vi "Phase array Simulation(21.09.30_KJS).vi"() -> ()   [LabVIEW 2017]
uses:
  <vilib>/Analysis/3filter.llb/Filter Passband Type.ctl
  <vilib>/Analysis/baseanly.llb/Unit Vector (DBL).vi
  <vilib>/Analysis/2dsp.llb/Real FFT.vi
  <vilib>/Analysis/3filter.llb/FIR Windowed Filter (DBL).vi
  <vilib>/Analysis/NI_AALBase.lvlib
  <vilib>/Analysis/NI_AALPro.lvlib
panel:
  out "XY 그래프":cluster{dbl[], dbl[]}(graph)
  out "최대값":dbl
  in  "SNR(dB)":dbl=6.0
  out "doppler frequency % 2":dbl
  out "SUM signal(LPF)":waveform(dbl)(graph)
  out "S1+S3 signal(LPF)":waveform(dbl)(graph)
  out "S0+S2 signal(LPF)":waveform(dbl)(graph)
  out "Mixer(S1 +S3)":waveform(dbl)(graph)
  out "Mixer(S0 +S2)":waveform(dbl)(graph)
  out "S1+S3 FFT":waveform(dbl)(graph)
  out "S0+S2 FFT":waveform(dbl)(graph)
  out "S1+S3 signal":waveform(dbl)(graph)
  out "S0 +S2 signal":waveform(dbl)(graph)
  out "크기":i32
  in  "X(+)":bool
  in  "Delay time.A.1(sec)":dbl=0.5
  in  "Sampling frequency(Hz)":dbl=3000000.0
  in  "Pulse length(sec)":dbl=0.5
  in  "Amplitude(Vpeak)":dbl=1.0
  in  "Frequency(Hz)":dbl=614000.0
  in  "Carrier Frequency(Hz)":dbl=574000.0
  in  "S1+S3 Carrier Phsae":dbl=-90.0
  in  "S0+S2 Carrier Phsae":dbl=90.0
  in  "S0 Phsae":dbl=90.0
  in  "S1 Phsae":dbl=-90.0
  in  "S2 Phsae":dbl=-180.0
  in  "S3 Phsae":dbl=-270.0
  out "doppler frequency %":dbl
  in  "signal Dopphler On":bool
  in  "DpF":dbl=10000.0
  in  "Carrier Dopphler On":bool
  # "Signal Modeling Setting"
  # "Doppler shift Modeling Variable"
  # "Phase Modeling Variable"
  # "Simulation Button"
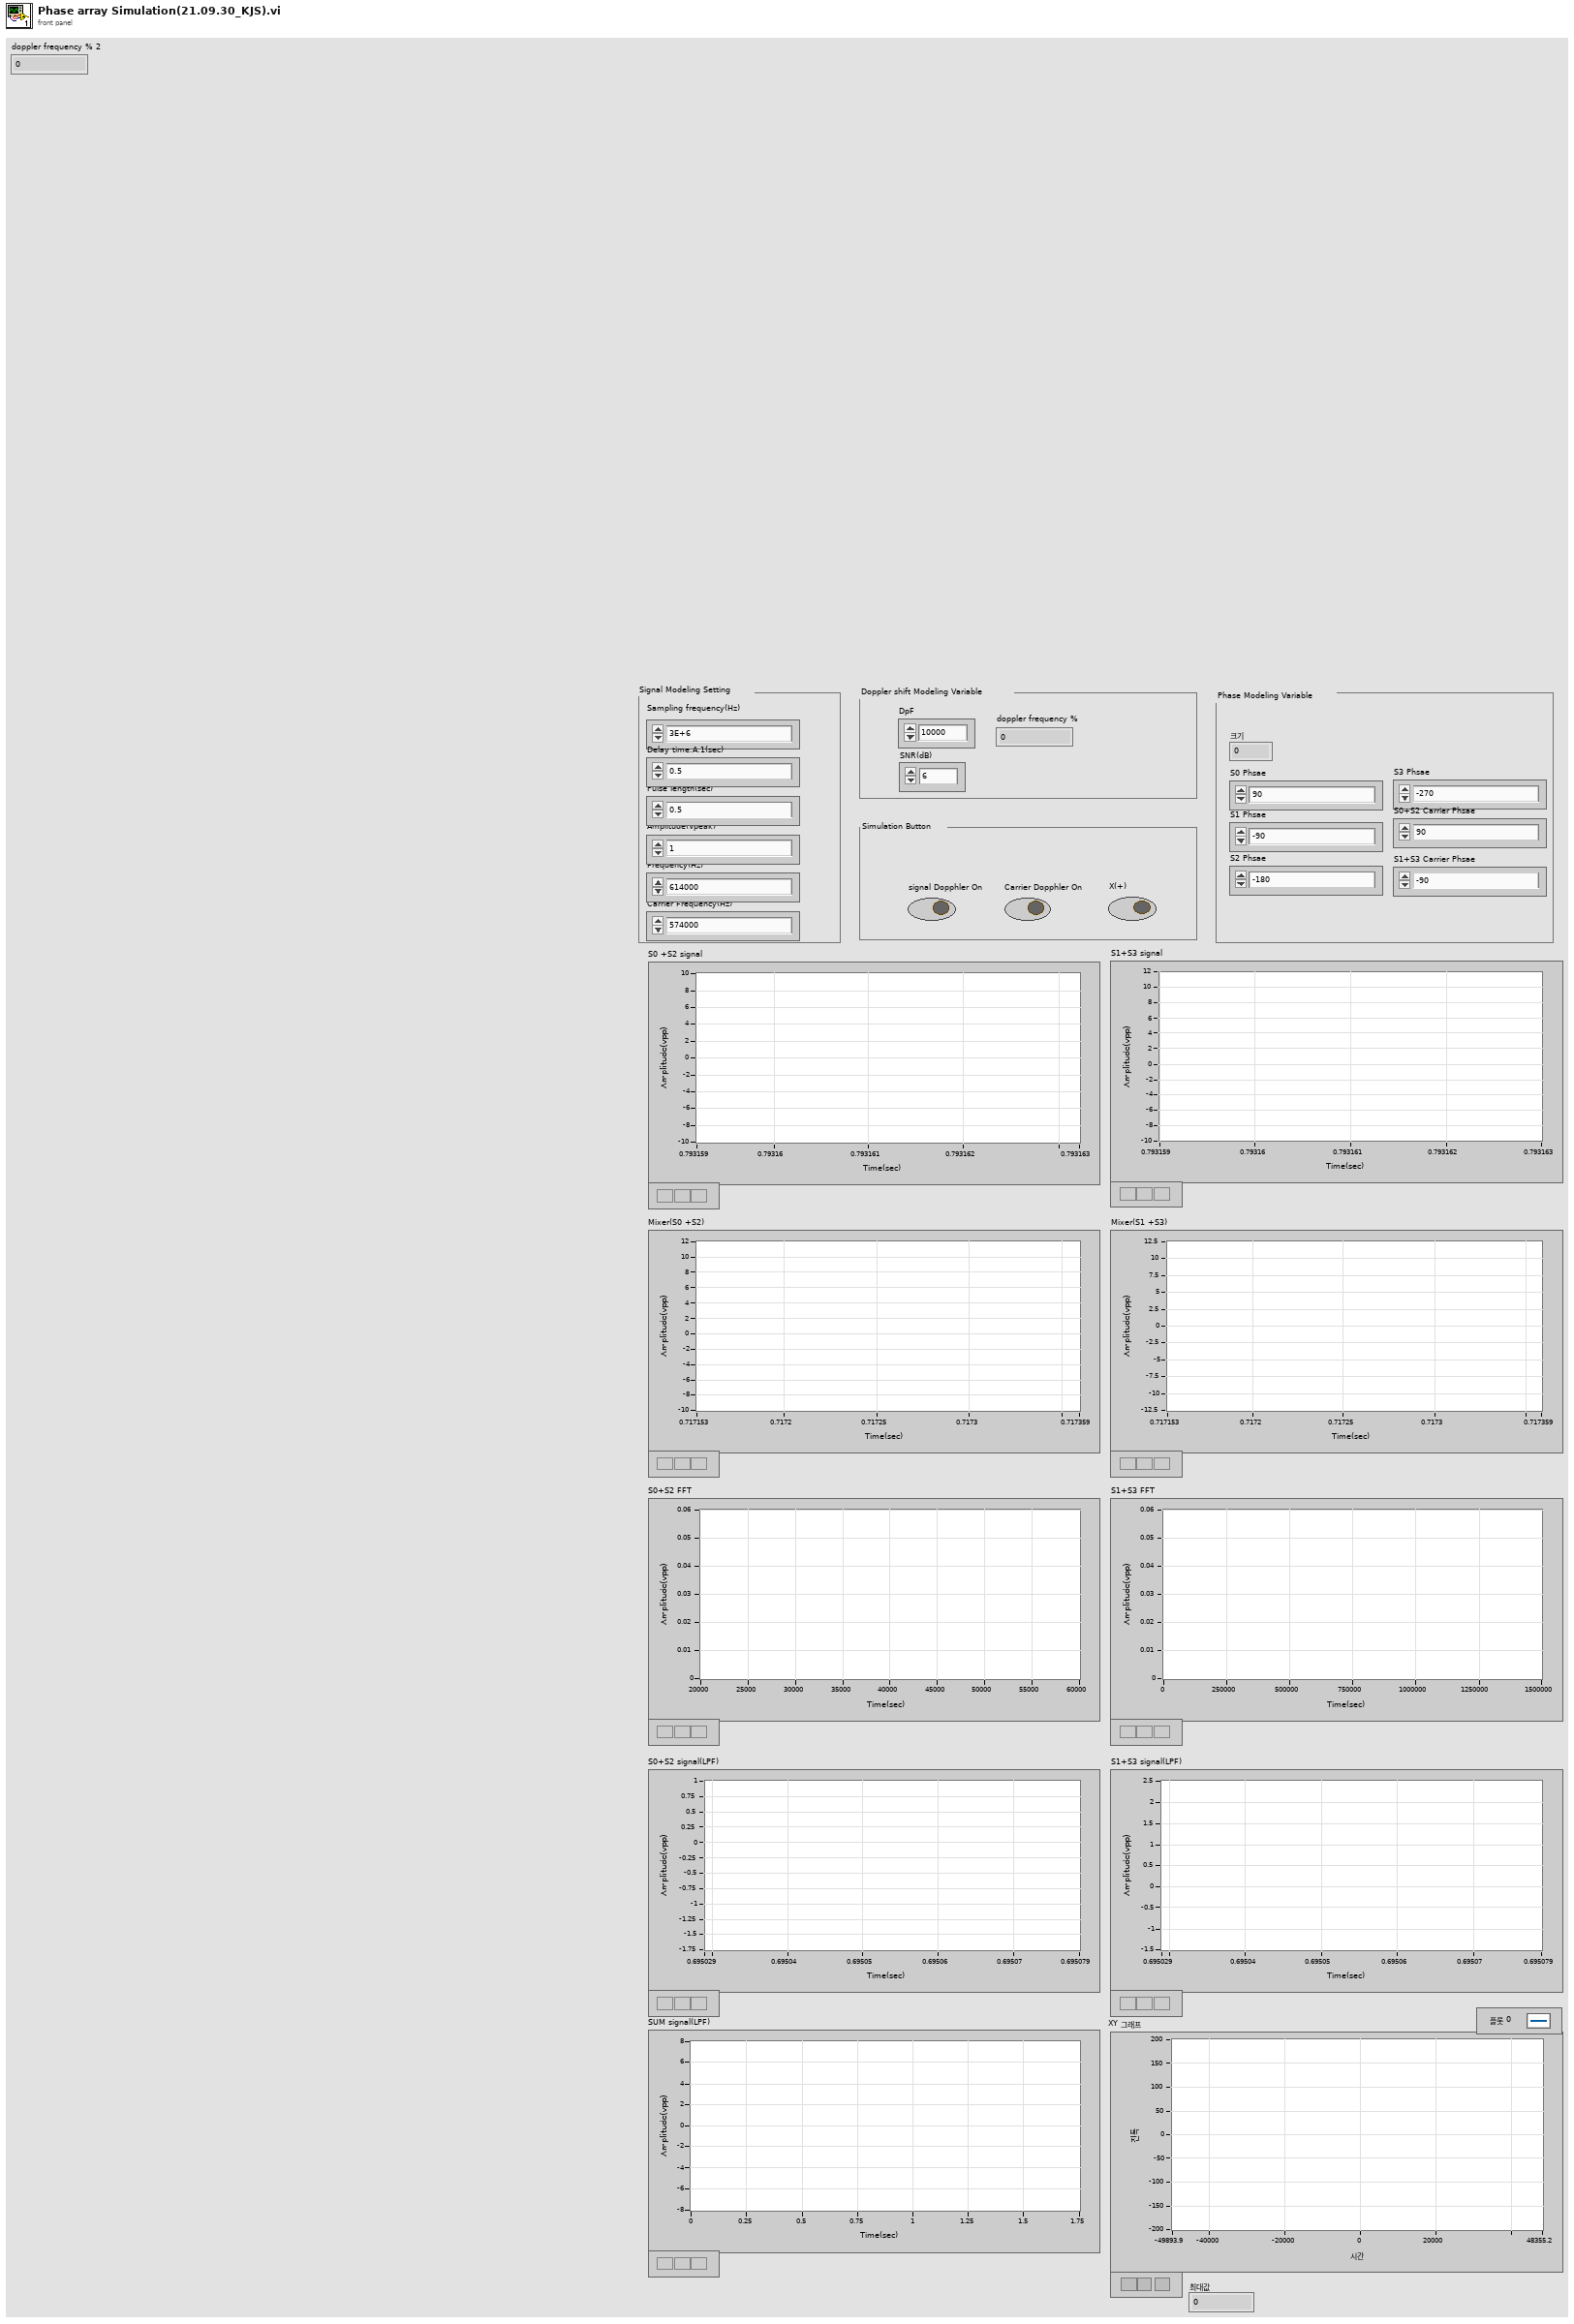
[diagram p1: front panel]
types:
  T1 = typedef "NI_AALBase.lvlib/Filter Passband Type.ctl" = enum32{"Lowpass", "Highpass", "Bandpass", "Bandstop"}
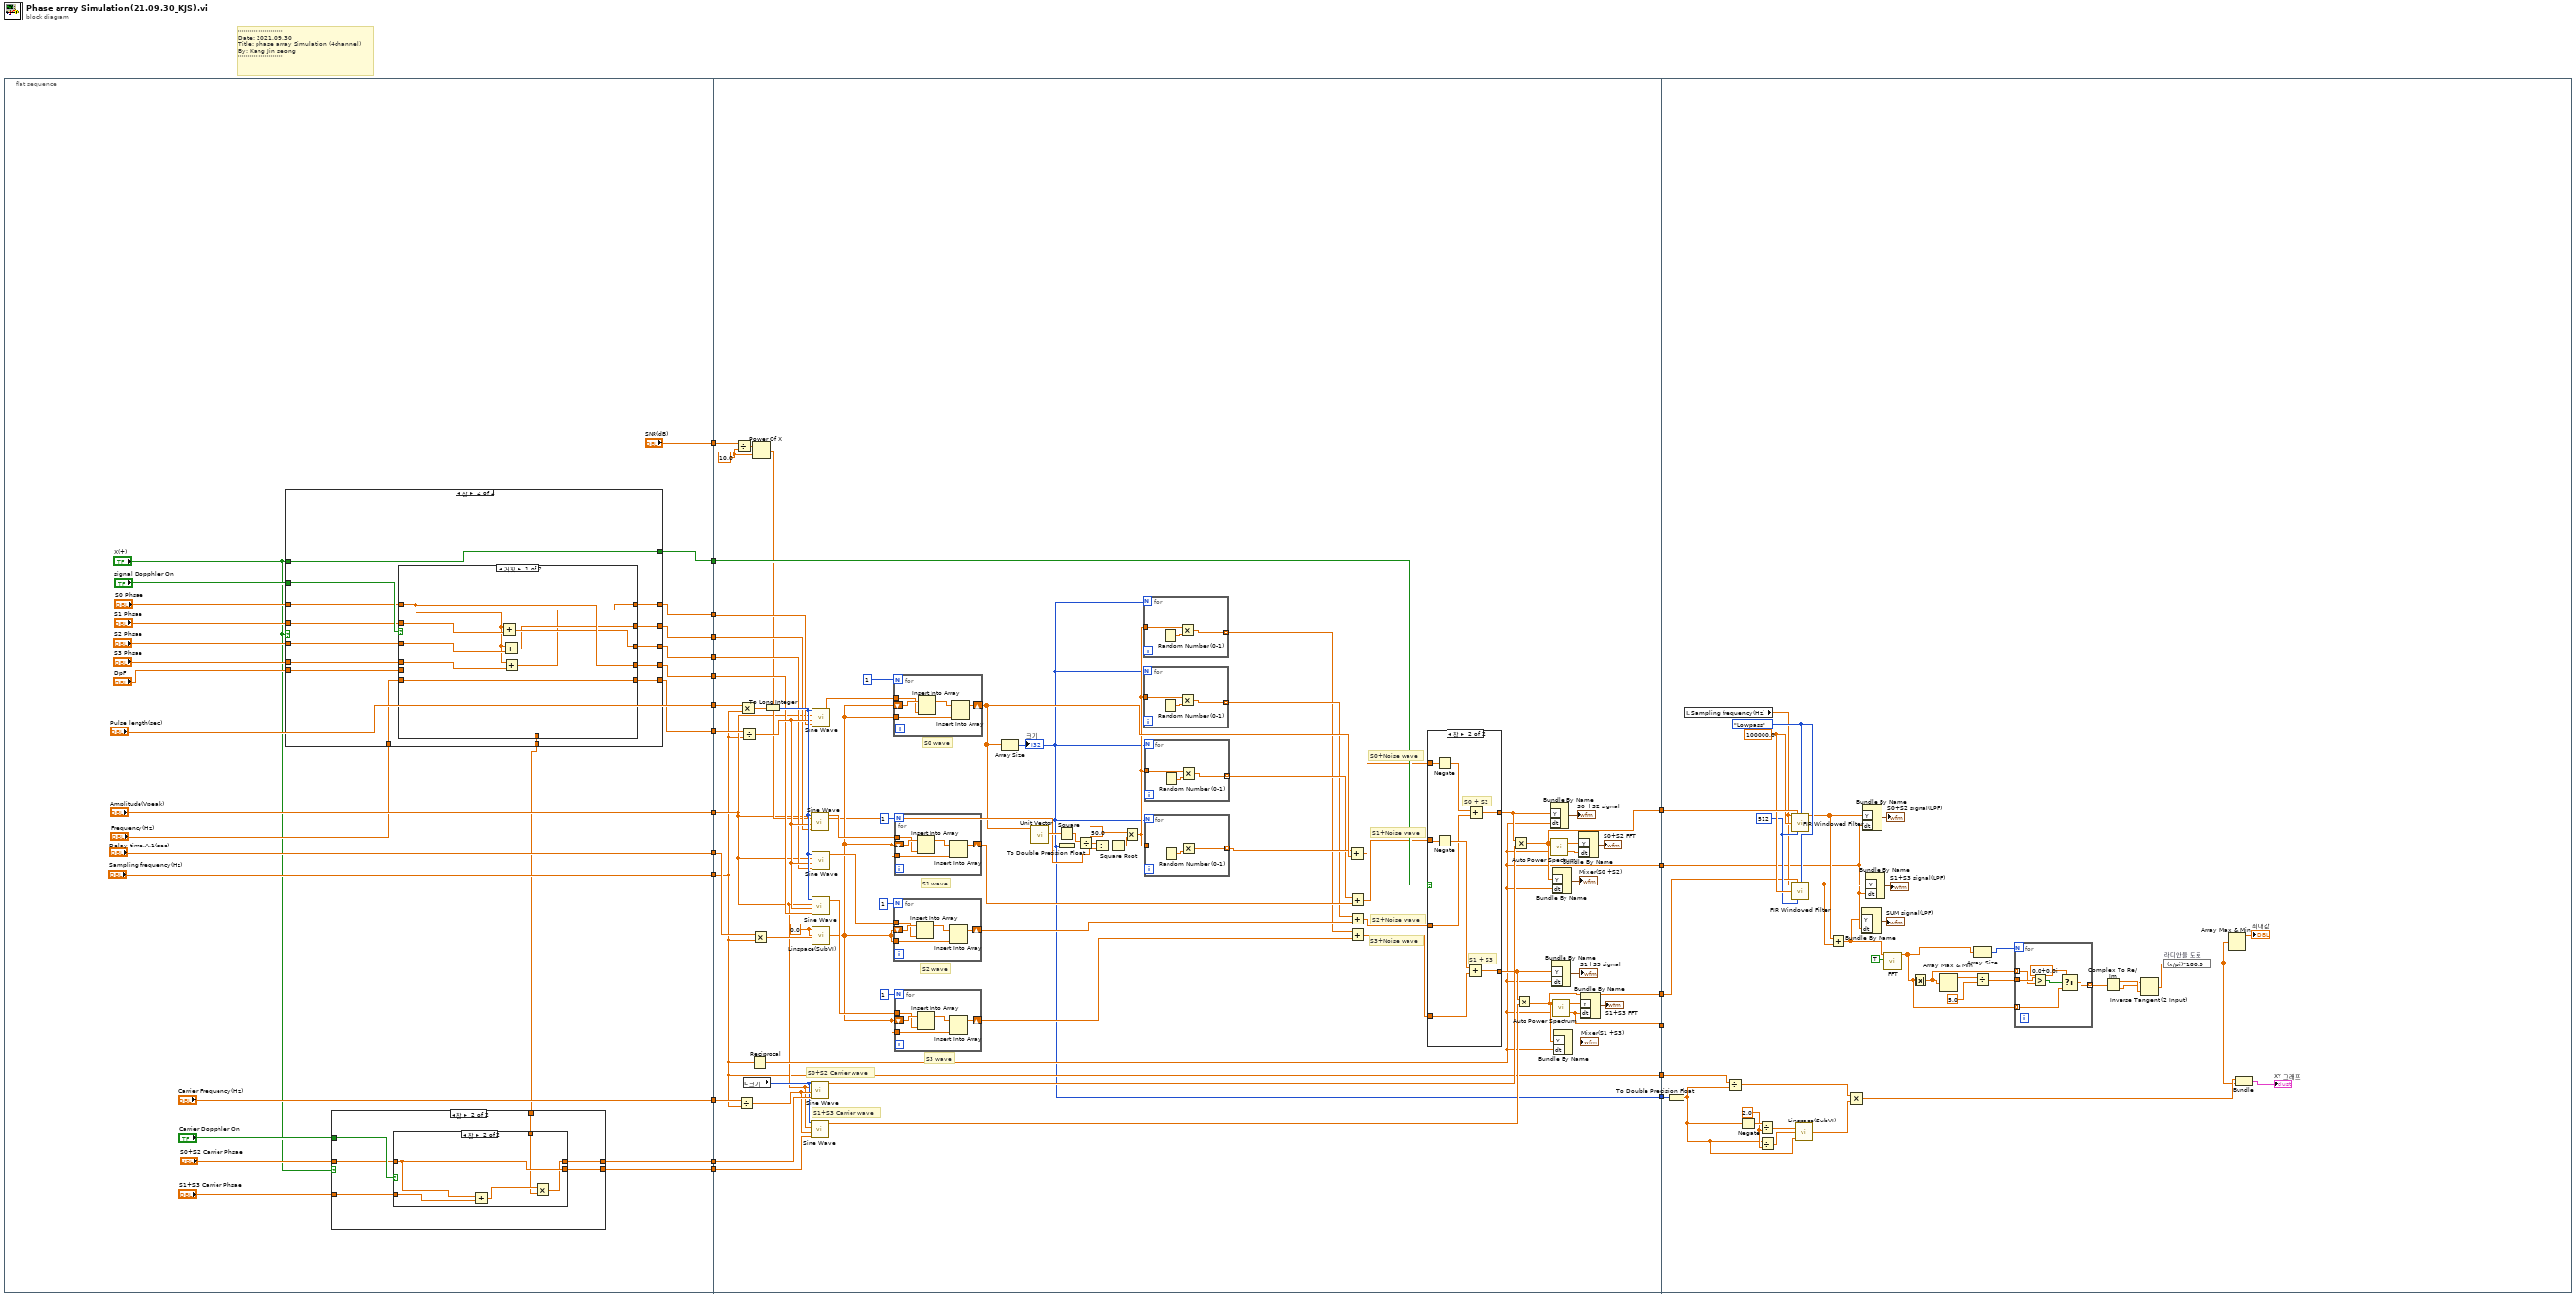
[diagram p0: block diagram]
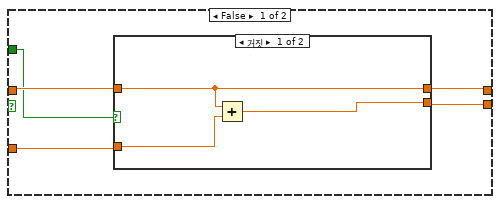
[diagram p2: hidden frame]
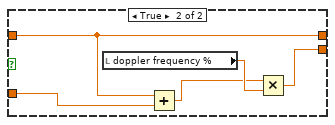
[diagram p3: hidden frame]
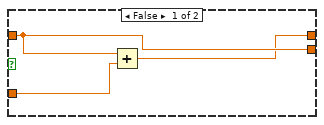
[diagram p4: hidden frame]
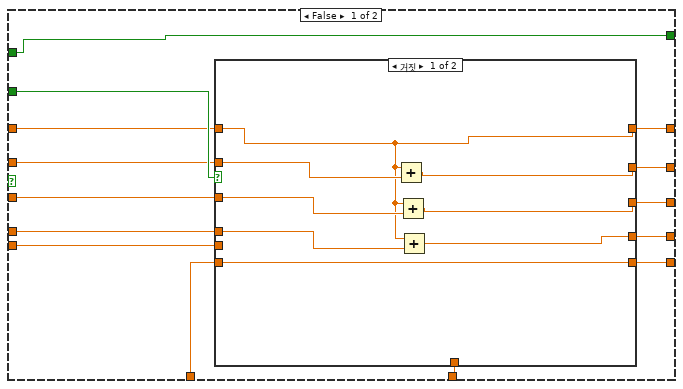
[diagram p5: hidden frame]
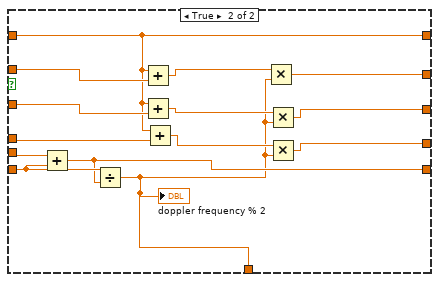
[diagram p6: hidden frame]
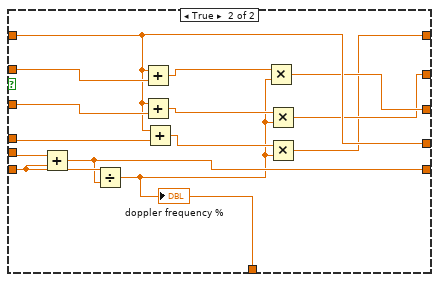
[diagram p7: hidden frame]
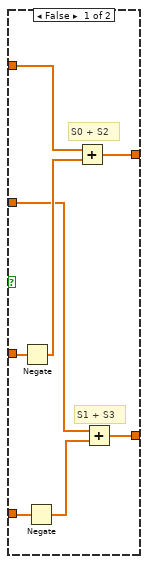
[diagram p8: hidden frame]
diagram:
  # "'''''''''''''''''''''''\nDate: 2021.09.30\nTitle: phase array Simulation (4channel)\nBy: Kang Jin seong\n'''''''''''''''''''''''"
  n1 = flat-sequence {
    tunnel: ["Carrier Frequency(Hz)"] -> w20
    tunnel: [w32] -> w19
    tunnel: ["Amplitude(Vpeak)"] -> w18
    tunnel: ["Pulse length(sec)"] -> w17
    tunnel: ["Sampling frequency(Hz)"] -> w16
    tunnel: ["Delay time.A.1(sec)"] -> w15
    tunnel: [w37] -> w14
    tunnel: [w36] -> w13
    tunnel: [w35] -> w12
    tunnel: [w34] -> w11
    tunnel: [w26] -> w10
    tunnel: [w25] -> w9
    tunnel: [w24] -> w5
    tunnel: ["SNR(dB)"] -> w4
    tunnel: w20 -> [w195]
    tunnel: w19 -> [w202]
    tunnel: w18 -> [w149]
    tunnel: w17 -> [w201]
    tunnel: w16 -> [w147]
    tunnel: w15 -> [w200]
    tunnel: w14 -> [w199]
    tunnel: w13 -> [w198]
    tunnel: w12 -> [w197]
    tunnel: w11 -> [w196]
    tunnel: w10 -> [w194]
    tunnel: w9 -> [w190]
    tunnel: [w178] -> w8
    tunnel: [w177] -> w7
    tunnel: [w176] -> w6
    tunnel: w5 -> [w175]
    tunnel: w4 -> [w172]
    tunnel: [w148] -> w3
    tunnel: [w147] -> w2
    tunnel: [w146] -> w1
    tunnel: w8 -> [w301]
    tunnel: w7 -> [w297]
    tunnel: w6 -> [w290]
    tunnel: w3 -> [_]
    tunnel: w2 -> [w277]
    tunnel: w1 -> [w276]
    frame #0 {
      n2 = case shown="참" "X(+)" {
        tunnel: "signal Dopphler On" -> [w86 w123]
        tunnel: "S0 Phsae" -> [w85 w122]
        tunnel: "S1 Phsae" -> [w84 w121]
        tunnel: "S2 Phsae" -> [w81 w120]
        tunnel: "S3 Phsae" -> [w80 w119]
        tunnel: [w79 w118] -> w37
        tunnel: [w78 w117] -> w36
        tunnel: [w77 w116] -> w35
        tunnel: [w76 w115] -> w34
        tunnel: "Frequency(Hz)" -> [w82 w114]
        tunnel: [w75 w113] -> w32
        tunnel: "DpF" -> [w83 w112]
        tunnel: [w87 w111] -> w24
        tunnel: "X(+)" -> [w87 w111]
        tunnel: [w74 w110] -> w21
        frame False {
          n3 = case shown="거짓" w86 {
            tunnel: w85 -> [w90 w99]
            tunnel: w84 -> [w94 w103]
            tunnel: w81 -> [w92 w101]
            tunnel: w80 -> [w89 w98]
            tunnel: [w90 w99] -> w79
            tunnel: [w93 w107] -> w78
            tunnel: [w91 w106] -> w77
            tunnel: [w88 w105] -> w76
            tunnel: w82 -> [w95 w108]
            tunnel: [w95 w104] -> w75
            tunnel: w83 -> [_ w109]
            tunnel: [_ w96] -> w74
            frame False {
              n4 = Add(x=w90, y=w94) -> (x+y=w93:dbl)
              n5 = Add(x=w90, y=w92) -> (x+y=w91:dbl)
              n6 = Add(x=w90, y=w89) -> (x+y=w88:dbl)
            }
            frame True {
              n7 = Add(x=w109, y=w108) -> (x+y=w104:dbl)
              n8 = Divide(x=w108, y=w104) -> (x/y=w96:dbl)
              "doppler frequency % 2" <- w96
              n9 = Add(x=w99, y=w103) -> (x+y=w102:dbl)
              n10 = Add(x=w99, y=w101) -> (x+y=w100:dbl)
              n11 = Add(x=w99, y=w98) -> (x+y=w97:dbl)
              n12 = Multiply(x=w102, y=w96) -> (x*y=w107:dbl)
              n13 = Multiply(x=w100, y=w96) -> (x*y=w106:dbl)
              n14 = Multiply(x=w97, y=w96) -> (x*y=w105:dbl)
            }
          }
        }
        frame True {
          n15 = case shown="거짓" w123 {
            tunnel: w122 -> [w127 w136]
            tunnel: w121 -> [w130 w142]
            tunnel: w120 -> [w129 w140]
            tunnel: w119 -> [w128 w138]
            tunnel: [w124 w133] -> w118
            tunnel: [w125 w134] -> w117
            tunnel: [w126 w135] -> w116
            tunnel: [w127 w136] -> w115
            tunnel: w114 -> [w131 w144]
            tunnel: [w131 w143] -> w113
            tunnel: w112 -> [_ w145]
            tunnel: [_ w132] -> w110
            frame False {
              n16 = Add(x=w127, y=w130) -> (x+y=w126:dbl)
              n17 = Add(x=w127, y=w129) -> (x+y=w125:dbl)
              n18 = Add(x=w127, y=w128) -> (x+y=w124:dbl)
            }
            frame True {
              n19 = Add(x=w145, y=w144) -> (x+y=w143:dbl)
              n20 = Divide(x=w144, y=w143) -> (x/y=w132:dbl)
              "doppler frequency %" <- w132
              n21 = Add(x=w136, y=w142) -> (x+y=w141:dbl)
              n22 = Add(x=w136, y=w140) -> (x+y=w139:dbl)
              n23 = Add(x=w136, y=w138) -> (x+y=w137:dbl)
              n24 = Multiply(x=w141, y=w132) -> (x*y=w135:dbl)
              n25 = Multiply(x=w139, y=w132) -> (x*y=w134:dbl)
              n26 = Multiply(x=w137, y=w132) -> (x*y=w133:dbl)
            }
          }
        }
      }
      n27 = case shown="참" "X(+)" {
        tunnel: "Carrier Dopphler On" -> [w47 w65]
        tunnel: "S0+S2 Carrier Phsae" -> [w51 w64]
        tunnel: "S1+S3 Carrier Phsae" -> [w50 w63]
        tunnel: [w49 w62] -> w26
        tunnel: [w48 w61] -> w25
        tunnel: w21 -> [_ w60]
        frame False {
          n28 = case shown="거짓" w47 {
            tunnel: w51 -> [w52 w55]
            tunnel: w50 -> [w54 w57]
            tunnel: [w52 w55] -> w49
            tunnel: [w53 w58] -> w48
            frame False {
              n29 = Add(x=w52, y=w54) -> (x+y=w53:dbl)
            }
            frame True {
              n30 = local read "doppler frequency %"() -> (w59:dbl)
              n31 = Add(x=w55, y=w57) -> (x+y=w56:dbl)
              n32 = Multiply(x=w56, y=w59) -> (x*y=w58:dbl)
            }
          }
        }
        frame True {
          n33 = case shown="참" w65 {
            tunnel: w64 -> [w67 w71]
            tunnel: w63 -> [w68 w73]
            tunnel: [w66 w70] -> w62
            tunnel: [w67 w71] -> w61
            tunnel: w60 -> [_ w69]
            frame False {
              n34 = Add(x=w67, y=w68) -> (x+y=w66:dbl)
            }
            frame True {
              n35 = Add(x=w71, y=w73) -> (x+y=w72:dbl)
              n36 = Multiply(x=w72, y=w69) -> (x*y=w70:dbl)
            }
          }
        }
      }
    }
    frame #1 {
      w174 = 10.0 ("y")
      w213 = 0.0 ("Start")
      # "S3+Noise wave"
      # "S2+Noise wave"
      # "S1+Noise wave"
      # "S0+Noise wave"
      # "S1+S3 Carrier wave"
      # "S0+S2 Carrier wave"
      # "S3 wave"
      # "S2 wave"
      # "S1 wave"
      # "S0 wave"
      n37 = Divide(x=w172, y=w174) -> (x/y=w173:dbl)
      n38 = Divide(x=w195, y=w147) -> (x/y=w191:dbl)
      n39 = Multiply(x=w201, y=w147) -> (x*y=w216:dbl)
      n40 = Divide(x=w202, y=w147) -> (x/y=w214:dbl)
      n41 = local read "크기"() -> (w150:i32)
      n42 = Reciprocal(x=w147) -> (1/x=w176:dbl)
      n43 = Multiply(x=w200, y=w147) -> (x*y=w212:dbl)
      n44 = Power Of X(1:w174, 2:w173) -> (0:w164:dbl)
      n45 = To Long Integer(number=w216) -> (32bit integer=w215:i32)
      n46 = call <vilib>:"Sine Wave.vi"("samples"=w150, "amplitude"=w149, "frequency"=w191, "phase in"=w194) -> ("sine wave"=w188:dbl[])  [unwired: 1 in, 2 out]
      n47 = call <vilib>:"Sine Wave.vi"("samples"=w215, "amplitude"=w149, "frequency"=w214, "phase in"=w198) -> ("sine wave"=w208:dbl[])  [unwired: 1 in, 2 out]
      n48 = call <vilib>:"Sine Wave.vi"("samples"=w150, "amplitude"=w149, "frequency"=w191, "phase in"=w190) -> ("sine wave"=w186:dbl[])  [unwired: 1 in, 2 out]
      n49 = call <vilib>:"Sine Wave.vi"("samples"=w215, "amplitude"=w149, "frequency"=w214, "phase in"=w196) -> ("sine wave"=w204:dbl[])  [unwired: 1 in, 2 out]
      n50 = call <vilib>:"Sine Wave.vi"("samples"=w215, "amplitude"=w149, "frequency"=w214, "phase in"=w199) -> ("sine wave"=w210:dbl[])  [unwired: 1 in, 2 out]
      n51 = call <vilib>:"Sine Wave.vi"("samples"=w215, "amplitude"=w149, "frequency"=w214, "phase in"=w197) -> ("sine wave"=w206:dbl[])  [unwired: 1 in, 2 out]
      n52 = call "Linspace(SubVI).vi"("NumElements"=w212, "End"=w213, "Start"=w213) -> ("Array"=w203:dbl[])
      n53 = for {
        N: 1 -> [_]
        shift-right: [w260] -> w163
        shift-left: w203 -> [w264]
        tunnel: w210 -> [w263]
        tunnel: w203 -> [w261]
        n54 = Insert Into Array(array=w264, new element=w263) -> (w262:dbl[])  [unwired: 1 in]
        n55 = Insert Into Array(array=w262, new element=w261) -> (w260:dbl[])  [unwired: 1 in]
      }
      n56 = for {
        N: 1 -> [_]
        shift-right: [w250] -> w161
        shift-left: w203 -> [w254]
        tunnel: w206 -> [w253]
        tunnel: w203 -> [w251]
        n57 = Insert Into Array(array=w254, new element=w253) -> (w252:dbl[])  [unwired: 1 in]
        n58 = Insert Into Array(array=w252, new element=w251) -> (w250:dbl[])  [unwired: 1 in]
      }
      n59 = for {
        N: 1 -> [_]
        shift-right: [w255] -> w162
        shift-left: w203 -> [w259]
        tunnel: w208 -> [w258]
        tunnel: w203 -> [w256]
        n60 = Insert Into Array(array=w259, new element=w258) -> (w257:dbl[])  [unwired: 1 in]
        n61 = Insert Into Array(array=w257, new element=w256) -> (w255:dbl[])  [unwired: 1 in]
      }
      n62 = for {
        N: 1 -> [_]
        shift-right: [w245] -> w160
        shift-left: w203 -> [w249]
        tunnel: w204 -> [w248]
        tunnel: w203 -> [w246]
        n63 = Insert Into Array(array=w249, new element=w248) -> (w247:dbl[])  [unwired: 1 in]
        n64 = Insert Into Array(array=w247, new element=w246) -> (w245:dbl[])  [unwired: 1 in]
      }
      n65 = Array Size(array=w163) -> (size(s)=w146:i32)
      "크기" <- w146
      n66 = call-poly <vilib>:"Unit Vector.vi"("Input Vector"=w163) -> ("norm"=w171:dbl)  [unwired: 8 in, 2 out]
      n67 = Square(x=w171) -> (x^2=w170:dbl)
      n68 = To Double Precision Float(number=w146) -> (double precision float=w169:dbl)
      n69 = Divide(x=w170, y=w169) -> (x/y=w168:dbl)
      n70 = Divide(x=w168, y=w164) -> (x/y=w167:dbl)
      n71 = Square Root(x=w167) -> (sqrt(x)=w166:dbl)
      n72 = Multiply(x=50.0, y=w166) -> (x*y=w159:dbl)
      n73 = for {
        N: w146 -> [_]
        tunnel: w159 -> [w218]
        tunnel: [w217] -> w155 mode=indexing
        n74 = Random Number (0-1)() -> (number: 0 to 1=w219:dbl)
        n75 = Multiply(x=w218, y=w219) -> (x*y=w217:dbl)
      }
      n76 = for {
        N: w146 -> [_]
        tunnel: w159 -> [w221]
        tunnel: [w220] -> w156 mode=indexing
        n77 = Random Number (0-1)() -> (number: 0 to 1=w222:dbl)
        n78 = Multiply(x=w221, y=w222) -> (x*y=w220:dbl)
      }
      n79 = for {
        N: w146 -> [_]
        tunnel: w159 -> [w224]
        tunnel: [w223] -> w157 mode=indexing
        n80 = Random Number (0-1)() -> (number: 0 to 1=w225:dbl)
        n81 = Multiply(x=w224, y=w225) -> (x*y=w223:dbl)
      }
      n82 = for {
        N: w146 -> [_]
        tunnel: w159 -> [w227]
        tunnel: [w226] -> w158 mode=indexing
        n83 = Random Number (0-1)() -> (number: 0 to 1=w228:dbl)
        n84 = Multiply(x=w227, y=w228) -> (x*y=w226:dbl)
      }
      n85 = Add(x=w158, y=w163) -> (x+y=w154:dbl[])
      n86 = Add(x=w157, y=w162) -> (x+y=w153:dbl[])
      n87 = Add(x=w156, y=w161) -> (x+y=w152:dbl[])
      n88 = Add(x=w155, y=w160) -> (x+y=w151:dbl[])
      n89 = case shown="참" w175 {
        tunnel: w154 -> [w235 w240]
        tunnel: w152 -> [w236 w237]
        tunnel: w153 -> [w232 w244]
        tunnel: w151 -> [w233 w242]
        tunnel: [w230 w239] -> w189
        tunnel: [w229 w241] -> w187
        frame False {
          # "S1 + S3"
          # "S0 + S2"
          n90 = Negate(x=w236) -> (-x=w234:dbl[])
          n91 = Negate(x=w233) -> (-x=w231:dbl[])
          n92 = Add(x=w235, y=w234) -> (x+y=w230:dbl[])
          n93 = Add(x=w232, y=w231) -> (x+y=w229:dbl[])
        }
        frame True {
          # "S1 + S3"
          # "S0 + S2"
          n94 = Negate(x=w240) -> (-x=w238:dbl[])
          n95 = Negate(x=w244) -> (-x=w243:dbl[])
          n96 = Add(x=w243, y=w242) -> (x+y=w241:dbl[])
          n97 = Add(x=w238, y=w237) -> (x+y=w239:dbl[])
        }
      }
      n98 = Multiply(x=w189, y=w188) -> (x*y=w178:dbl[])
      n99 = Multiply(x=w187, y=w186) -> (x*y=w177:dbl[])
      n100 = Bundle By Name("Y"=w189, "dt"=w176) -> (→"S0 +S2 signal":waveform(dbl))  [unwired: 1 in]
      n101 = call <vilib>:"Auto Power Spectrum.vi"("dt"=w176, "Signal (V)"=w178) -> ("df"=w183:dbl, "Power Spectrum (V^2 rms)"=w184:dbl[])
      n102 = Bundle By Name("Y"=w187, "dt"=w176) -> (→"S1+S3 signal":waveform(dbl))  [unwired: 1 in]
      n103 = Bundle By Name("Y"=w178, "dt"=w176) -> (→"Mixer(S0 +S2)":waveform(dbl))  [unwired: 1 in]
      n104 = call <vilib>:"Auto Power Spectrum.vi"("dt"=w176, "Signal (V)"=w177) -> ("df"=w148:dbl, "Power Spectrum (V^2 rms)"=w181:dbl[])
      n105 = Bundle By Name("Y"=w177, "dt"=w176) -> (→"Mixer(S1 +S3)":waveform(dbl))  [unwired: 1 in]
      n106 = Bundle By Name("Y"=w184, "dt"=w183) -> (→"S0+S2 FFT":waveform(dbl))  [unwired: 1 in]
      n107 = Bundle By Name("Y"=w181, "dt"=w148) -> (→"S1+S3 FFT":waveform(dbl))  [unwired: 1 in]
    }
    frame #2 {
      w272 = 2.0 ("y")
      w298 = 512 ("taps")
      w299 = 100000.0 ("low cutoff freq: fl")
      w300 = Filter_Passband_Type."Lowpass" ("filter type")
      n108 = To Double Precision Float(number=w276) -> (double precision float=w269:dbl)
      n109 = local read "Sampling frequency(Hz)"() -> (w291:dbl)
      n110 = Divide(x=w277, y=w269) -> (x/y=w271:dbl)
      n111 = Negate(x=w269) -> (-x=w275:dbl)
      n112 = Divide(x=w275, y=w272) -> (x/y=w274:dbl)
      n113 = Divide(x=w269, y=w272) -> (x/y=w273:dbl)
      n114 = call-poly <vilib>:"FIR Windowed Filter.vi"("sampling freq: fs"=w291, "X"=w301, "filter type"=w300, "low cutoff freq: fl"=w299, "taps"=w298) -> ("Filtered X"=w294:dbl[])  [unwired: 9 in, 1 out]
      n115 = call-poly <vilib>:"FIR Windowed Filter.vi"("sampling freq: fs"=w291, "X"=w297, "filter type"=w300, "low cutoff freq: fl"=w299, "taps"=w298) -> ("Filtered X"=w293:dbl[])  [unwired: 9 in, 1 out]
      n116 = call "Linspace(SubVI).vi"("NumElements"=w269, "End"=w273, "Start"=w274) -> ("Array"=w270:dbl[])
      n117 = Add(x=w294, y=w293) -> (x+y=w289:dbl[])
      n118 = Multiply(x=w271, y=w270) -> (x*y=w268:dbl[])
      n119 = Bundle By Name("Y"=w289, "dt"=w290) -> (→"SUM signal(LPF)":waveform(dbl))  [unwired: 1 in]
      n120 = Bundle By Name("Y"=w294, "dt"=w290) -> (→"S0+S2 signal(LPF)":waveform(dbl))  [unwired: 1 in]
      n121 = Bundle By Name("Y"=w293, "dt"=w290) -> (→"S1+S3 signal(LPF)":waveform(dbl))  [unwired: 1 in]
      n122 = call-poly <vilib>:"FFT.vi"("shift?"=TRUE, "X"=w289) -> ("FFT {X}"=w283:cdb[])  [unwired: 8 in, 1 out]
      n123 = Absolute Value(x=w283) -> (abs(x)=w284:dbl[])
      n124 = Array Max & Min(array=w284) -> (max value=w288:dbl)  [unwired: 3 out]
      n125 = Array Size(array=w283) -> (size(s)=w286:i32)
      n126 = Divide(x=w288, y=5.0) -> (x/y=w285:dbl)
      n127 = for {
        N: w286 -> [_]
        tunnel: w285 -> [w307]
        tunnel: w284 -> [w306] mode=indexing
        tunnel: w283 -> [w303] mode=indexing
        tunnel: [w304] -> w282 mode=indexing
        n128 = Greater?(x=w307, y=w306) -> (0:w305:bool)
        n129 = Select(t=cdb 0.0+0.0i, s=w305, f=w303) -> (s? t:f=w304:cdb)
      }
      n130 = Complex To Re/Im(x + iy=w282) -> (x=w281:dbl[], y=w280:dbl[])
      n131 = Inverse Tangent (2 Input)(1:w281, 2:w280) -> (0:w267:dbl[])
      n132 = expression code="(x/pi)*180.0" "라디안을 도로"(w267) -> (w265:dbl[])
      n133 = Array Max & Min(array=w265) -> (max value=→"최대값":dbl)  [unwired: 3 out]
      n134 = Bundle(w268, w265) -> (→"XY 그래프":cluster{dbl[], dbl[]})  [unwired: 1 in]
    }
  }
